vi "poly_linspace_CXT.vi"(6 "inclusive? (T)":bool=TRUE, 7 "mode (cartesian)":T1(ring), 8 "xN":cxt, 9 "N":i32, 10 "x0":cxt) -> (1 "linspace out":cxt[](array[numeric]))   [LabVIEW 2015]
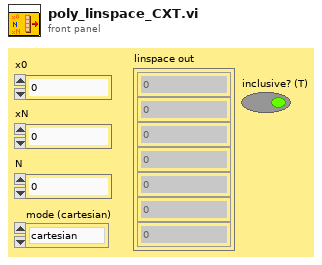
[diagram p1: front panel]
types:
  T1 = enum16{"cartesian", "angular (+)", "angular (-)"}
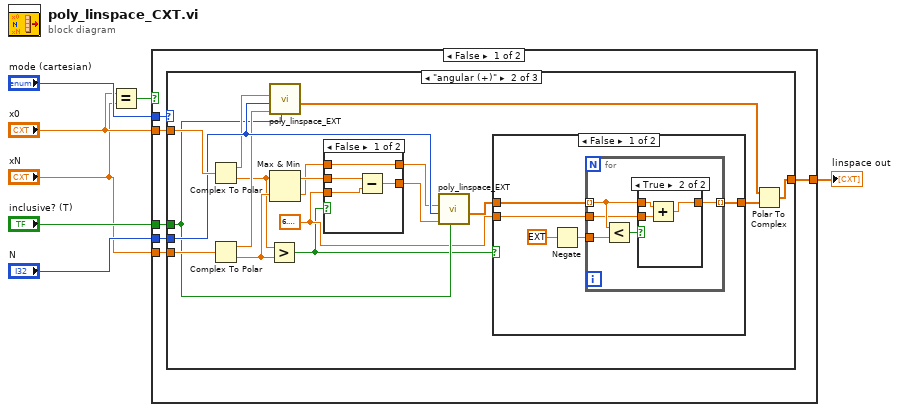
[diagram p0: block diagram]
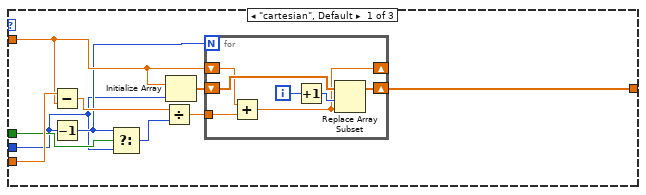
[diagram p2: hidden frame]
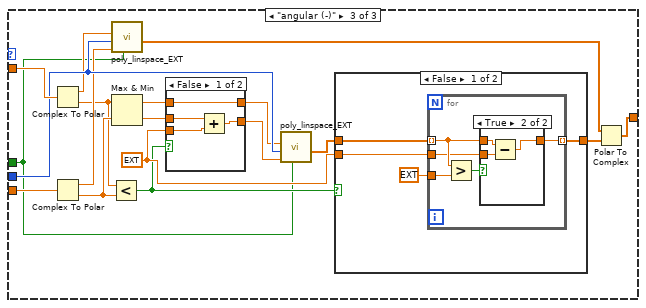
[diagram p6: hidden frame]
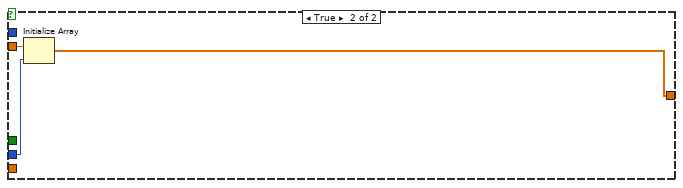
[diagram p10: hidden frame]
diagram:
  n1 = Equal?(x="x0", y="xN") -> (x = y?=w1:bool)
  n2 = case shown="False" w1 {
    tunnel: "xN" -> [w13 _]
    tunnel: "x0" -> [w12 w110]
    tunnel: "inclusive? (T)" -> [w11 _]
    tunnel: "N" -> [w10 w109]
    tunnel: [w9 w108] -> w5
    tunnel: "mode (cartesian)" -> [w8 _]
    frame False {
      n3 = case shown="\"angular (+)\"" w8 {
        tunnel: [w22 w44 w83] -> w9
        tunnel: w13 -> [w21 w47 w86]
        tunnel: w12 -> [w20 w48 w87]
        tunnel: w11 -> [w18 w38 w70]
        tunnel: w10 -> [w14 w46 w85]
        frame "cartesian", Default {
          n4 = Subtract(x=w21, y=w20) -> (x-y=w16:cxt)
          n5 = Decrement(x=w14) -> (x-1=w15:i32)
          n6 = Select(t=w15, s=w18, f=w14) -> (s? t:f=w17:i32)
          n7 = Divide(x=w16, y=w17) -> (x/y=w19:cxt)
          n8 = Initialize Array(w20, w14) -> (w23:cxt[])
          n9 = for {
            N: w15 -> [_]
            shift-right: [w27] -> w22
            shift-left: w23 -> [w30]
            shift-right: [w24] -> _
            shift-left: w20 -> [w29]
            tunnel: w19 -> [w28]
            i -> [w26]
            n10 = Add(x=w29, y=w28) -> (x+y=w24:cxt)
            n11 = Increment(x=w26) -> (x+1=w25:i32)
            n12 = Replace Array Subset(array=w30, new element=w24, index=w25) -> (w27:cxt[])
          }
        }
        frame "angular (+)" {
          w32 = 6.283185307179586
          n13 = Complex To Polar(r * e^(i*theta)=w48) -> (r=w43:ext, theta=w39:ext)
          n14 = Complex To Polar(r * e^(i*theta)=w47) -> (r=w42:ext, theta=w40:ext)
          n15 = Greater?(x=w39, y=w40) -> (0:w31:bool)
          n16 = call "poly_linspace_EXT.vi"("inclusive? (T)"=w38, "xN"=w42, "N"=w46, "x0"=w43) -> ("linspace out"=w45:ext[])  [unwired: 7 in]
          n17 = Max & Min(x=w39, y=w40) -> (max(x,y)=w37:ext, min(x,y)=w34:ext)
          n18 = case shown="False" w31 {
            tunnel: w37 -> [w66 w69]
            tunnel: [w67 w69] -> w36
            tunnel: [w65 w68] -> w35
            tunnel: w34 -> [w67 w68]
            tunnel: w32 -> [w64 _]
            frame False {
              n19 = Subtract(x=w66, y=w64) -> (x-y=w65:ext)
            }
            frame True {
            }
          }
          n20 = call "poly_linspace_EXT.vi"("inclusive? (T)"=w38, "xN"=w35, "N"=w46, "x0"=w36) -> ("linspace out"=w33:ext[])  [unwired: 7 in]
          n21 = case shown="False" w31 {
            tunnel: [w52 w63] -> w41
            tunnel: w33 -> [w53 w63]
            tunnel: w32 -> [w51 _]
            frame False {
              n22 = Negate(x=ext 3.1415926535897932385) -> (-x=w49:ext)
              n23 = for {
                tunnel: w53 -> [w56] mode=indexing
                tunnel: [w57] -> w52 mode=indexing
                tunnel: w51 -> [w55]
                tunnel: w49 -> [w54]
                n24 = Less?(x=w56, y=w54) -> (x < y?=w58:bool)
                n25 = case shown="True" w58 {
                  tunnel: [w59 w60] -> w57
                  tunnel: w56 -> [w59 w62]
                  tunnel: w55 -> [_ w61]
                  frame False {
                  }
                  frame True {
                    n26 = Add(x=w62, y=w61) -> (x+y=w60:ext)
                  }
                }
              }
            }
            frame True {
            }
          }
          n27 = Polar To Complex(1:w41, 2:w45) -> (0:w44:cxt[])
        }
        frame "angular (-)" {
          w72 = ext 6.283185307179586477
          n28 = Complex To Polar(r * e^(i*theta)=w87) -> (r=w82:ext, theta=w78:ext)
          n29 = Complex To Polar(r * e^(i*theta)=w86) -> (r=w81:ext, theta=w79:ext)
          n30 = Less?(x=w78, y=w79) -> (x < y?=w71:bool)
          n31 = call "poly_linspace_EXT.vi"("inclusive? (T)"=w70, "xN"=w81, "N"=w85, "x0"=w82) -> ("linspace out"=w84:ext[])  [unwired: 7 in]
          n32 = Max & Min(x=w78, y=w79) -> (max(x,y)=w77:ext, min(x,y)=w74:ext)
          n33 = case shown="False" w71 {
            tunnel: w77 -> [w103 w106]
            tunnel: [w103 w107] -> w76
            tunnel: [w105 w106] -> w75
            tunnel: w74 -> [w102 w107]
            tunnel: w72 -> [w104 _]
            frame False {
              n34 = Add(x=w102, y=w104) -> (x+y=w105:ext)
            }
            frame True {
            }
          }
          n35 = call "poly_linspace_EXT.vi"("inclusive? (T)"=w70, "xN"=w75, "N"=w85, "x0"=w76) -> ("linspace out"=w73:ext[])  [unwired: 7 in]
          n36 = case shown="False" w71 {
            tunnel: [w90 w101] -> w80
            tunnel: w73 -> [w91 w101]
            tunnel: w72 -> [w89 _]
            frame False {
              n37 = for {
                tunnel: w91 -> [w94] mode=indexing
                tunnel: [w95] -> w90 mode=indexing
                tunnel: w89 -> [w93]
                tunnel: ext 3.1415926535897932385 -> [w92]
                n38 = Greater?(x=w94, y=w92) -> (0:w96:bool)
                n39 = case shown="True" w96 {
                  tunnel: [w97 w98] -> w95
                  tunnel: w94 -> [w97 w100]
                  tunnel: w93 -> [_ w99]
                  frame False {
                  }
                  frame True {
                    n40 = Subtract(x=w100, y=w99) -> (x-y=w98:ext)
                  }
                }
              }
            }
            frame True {
            }
          }
          n41 = Polar To Complex(1:w80, 2:w84) -> (0:w83:cxt[])
        }
      }
    }
    frame True {
      n42 = Initialize Array(w110, w109) -> (w108:cxt[])
    }
  }
  "linspace out" <- w5
